vi "GPIB query.vi"(0 "address string":string, 1 "data":string, 2 "byte count":i32, 3 "error in":errorcluster, 4 "reading \nmode (0)":i16) -> (5 "data 2":string, 6 "error out (read)":errorcluster)   [LabVIEW 2017]
uses:
  <vilib>/Instr/_visa.llb/GPIB Status Boolean Array.ctl
panel:
  out "error out (write)":errorcluster
  out "ibsta 2":T1
  out "ibsta":T1
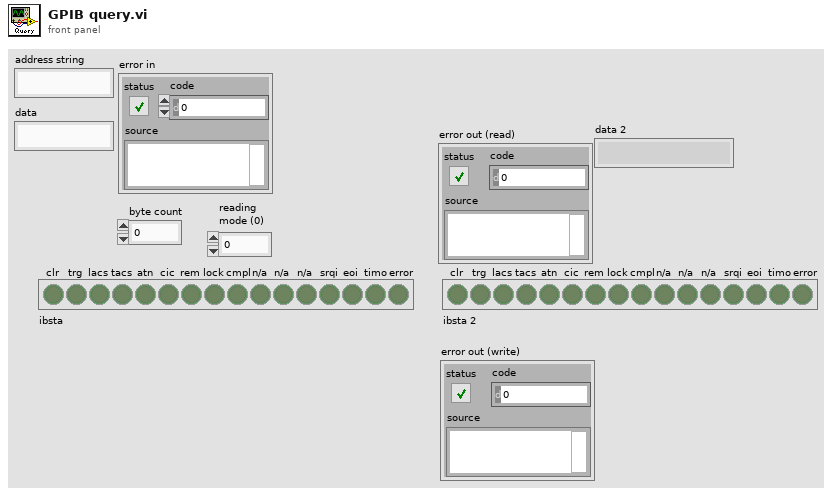
[diagram p1: front panel]
types:
  T1 = typedef "GPIB Status Boolean Array.ctl" = bool[]
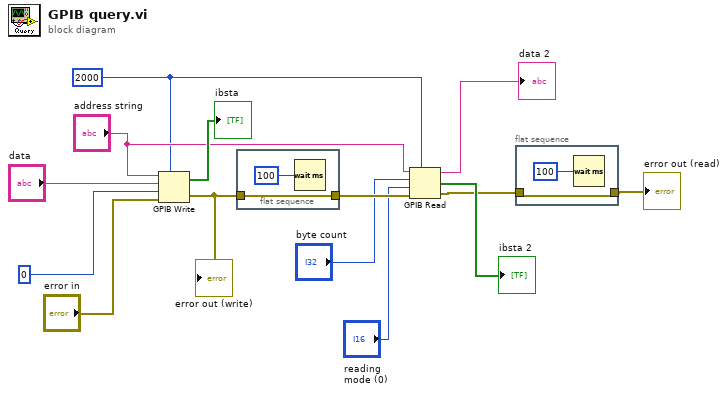
[diagram p0: block diagram]
diagram:
  w5 = 2000 ("timeout ms (488.2 global)")
  n1 = GPIB Write(0:"address string", 1:"data", 2:i16 0 ("mode (0)"), 3:"error in", 4:w5) -> (5:→"ibsta":bool[], 6:w14:errorcluster)
  "error out (write)" <- w14
  n2 = flat-sequence {
    tunnel: w14 -> [w16]
    tunnel: [w16] -> w13
    frame #0 {
      n3 = Wait (ms)(milliseconds to wait=u32 100) -> ()  [unwired: 1 out]
    }
  }
  n4 = GPIB Read(0:"address string", 1:"byte count", 2:"reading \nmode (0)", 3:w13, 4:w5) -> (5:→"data 2":string, 6:→"ibsta 2":bool[], 7:w2:errorcluster)
  n5 = flat-sequence {
    tunnel: w2 -> [w17]
    tunnel: [w17] -> w1
    frame #0 {
      n6 = Wait (ms)(milliseconds to wait=u32 100) -> ()  [unwired: 1 out]
    }
  }
  "error out (read)" <- w1
